vi "Write Component Path.vi"(8 "error in (no error)":errorcluster, 10 "Component's Path":path, 11 "Component in":refnum<class "Component.lvclass">) -> (0 "error out":errorcluster, 3 "Component out":refnum<class "Component.lvclass">)   [LabVIEW 2017, in "CL_G3_VIComponentBuilder.lvlib" / "Component.lvclass"]
uses:
  Component.lvclass
  Component.lvclass/Component.ctl
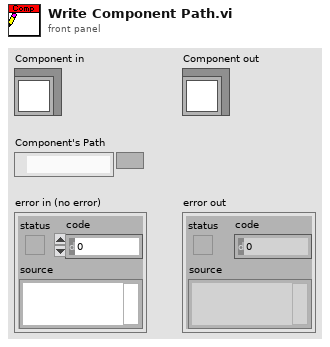
[diagram p1: front panel]
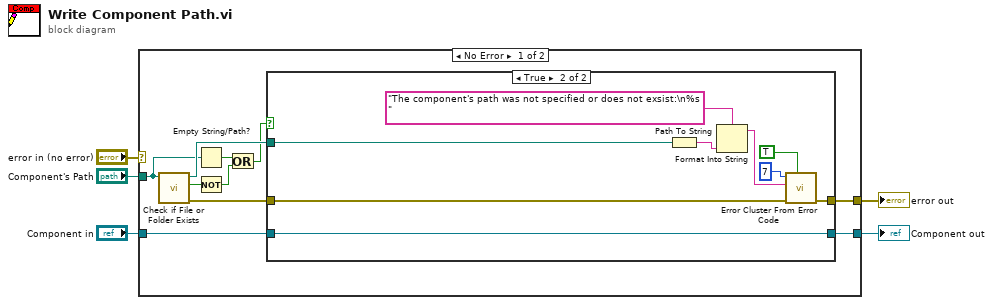
[diagram p0: block diagram]
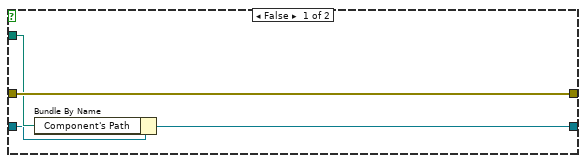
[diagram p2: hidden frame]
diagram:
  n1 = case shown="No Error" "error in (no error)" {
    selector: "error in (no error)" -> [_ w29]
    tunnel: [w6 w29] -> w1
    tunnel: [w7 w30] -> w3
    tunnel: "Component in" -> [w8 w30]
    tunnel: "Component's Path" -> [w9 _]
    frame No Error {
      n2 = call <vilib>:"Check if File or Folder Exists.vi"("path"=w9) -> ("error out"=w14:errorcluster, "file or folder exists?"=w13:bool, "dup path"=w15:path)  [unwired: 8 in]
      n3 = Empty String/Path?(string/path=w9) -> (empty?=w10:bool)
      n4 = Not(x=w13) -> (.not. x?=w12:bool)
      n5 = Or(x=w10, y=w12) -> (x .or. y?=w11:bool)
      n6 = case shown="True" w11 {
        tunnel: w8 -> [w17 w28]
        tunnel: [w16 w28] -> w7
        tunnel: w15 -> [w18 w27]
        tunnel: [w19 w20] -> w6
        tunnel: w14 -> [w19 w21]
        frame False {
          n7 = Bundle By Name(cluster=w17, "Component's Path"=w18) -> (w16:refnum<class "Component.lvclass">)
        }
        frame True {
          n8 = Path To String(path=w27) -> (string=w26:string)
          n9 = Format Into String(format string="The component's path was not specified or does not exsist:\n%s ", w26) -> (resulting string=w22:string)  [unwired: 2 in, 1 out]
          n10 = call <vilib>:"Error Cluster From Error Code.vi"("show call chain? (False)"=TRUE, "error in (no error)"=w21, "error message (\"\")"=w22, "error code (0)"=7) -> ("error out"=w20:errorcluster)  [unwired: 5 in]
        }
      }
    }
    frame Error {
    }
  }
  "error out" <- w1
  "Component out" <- w3
